vi "subDAQ_GetSnapPoint.vi"(5 "Record Table Refnum":refnum<vi>, 7 "Snap Number Refnum":refnum<vi>, 8 "Snap Point Y Arr Refnum":refnum<vi>, 9 "Snap Point X Arr Refnum":refnum<vi>, 10 "Snap Number Counting":dbl=2.0, 11 "Stage Status":T1={" Current Position"=[4.5511, -4.228, 0.0], "Number of Axis"=3, "ILSID"=1}) -> (1 "Snap Point cluster":cluster{"Snap Y":dbl[], "Snap X":dbl[]}={"Snap Y"=[-4.228, -2.7513], "Snap X"=[4.5511, 4.6806]}, 2 "Snap Point  Y Array":dbl[](array[numeric]), 3 "Snap Point  X Array":dbl[](array[numeric]))   [LabVIEW 2015]
panel:
  # "X"
  # "Y"
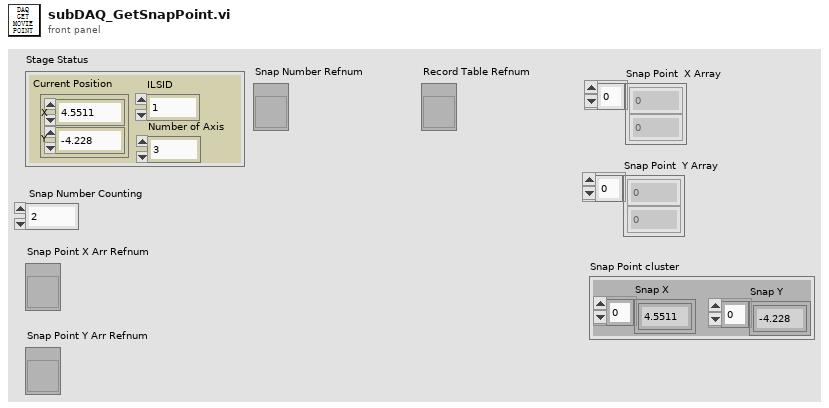
[diagram p1: front panel]
types:
  T1 = cluster{" Current Position":dbl[], "Number of Axis":i32, "ILSID":i32}
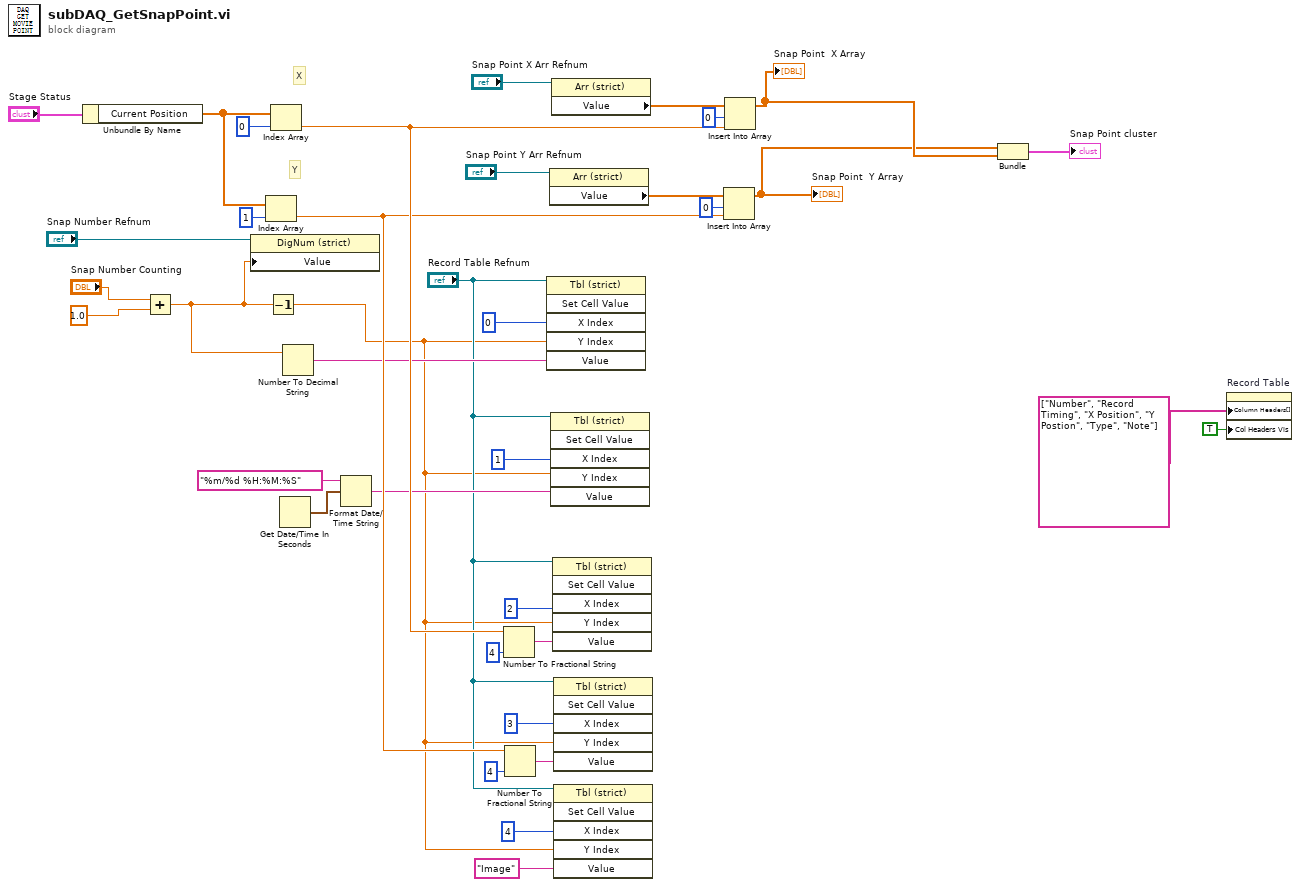
[diagram p0: block diagram]
diagram:
  # "Y"
  # "X"
  n1 = Unbundle By Name("Stage Status") -> ("Current Position"=w23:dbl[])
  n2 = Add(x="Snap Number Counting", y=1.0) -> (x+y=w4:dbl)
  n3 = property class="DigNum (strict)"(reference="Snap Number Refnum", "Value"=w4) -> ()  [unwired: 1 in, 2 out]
  n4 = Index Array(array=w23, index=1) -> (element=w26:dbl)
  n5 = Decrement(x=w4) -> (x-1=w3:dbl)
  n6 = Index Array(array=w23, index=0) -> (element=w27:dbl)
  n7 = Get Date/Time In Seconds() -> (seconds since 1Jan1904=w30:timestamp)
  n8 = Number To Decimal String(number=w4) -> (decimal integer string=w14:string)  [unwired: 1 in]
  n9 = Format Date/Time String(time format string (%c)="%m/%d %H:%M:%S", seconds (now)=w30) -> (date/time string=w12:string)  [unwired: 1 in]
  n10 = Number To Fractional String(number=w27, precision (6)=i16 4) -> (F-format string=w10:string)  [unwired: 2 in]
  n11 = Number To Fractional String(number=w26, precision (6)=i16 4) -> (F-format string=w8:string)  [unwired: 2 in]
  n12 = invoke class="Tbl (strict)" method="Set Cell Value"(reference="Record Table Refnum", "X Index"=0, "Y Index"=w3, "Value"=w14) -> ()  [unwired: 2 in, 6 out]
  n13 = property class="Arr (strict)"(reference="Snap Point Y Arr Refnum") -> ("Value"=w16:dbl[])  [unwired: 1 in, 2 out]
  n14 = invoke class="Tbl (strict)" method="Set Cell Value"(reference="Record Table Refnum", "X Index"=1, "Y Index"=w3, "Value"=w12) -> ()  [unwired: 2 in, 6 out]
  n15 = property class="Arr (strict)"(reference="Snap Point X Arr Refnum") -> ("Value"=w18:dbl[])  [unwired: 1 in, 2 out]
  n16 = invoke class="Tbl (strict)" method="Set Cell Value"(reference="Record Table Refnum", "X Index"=2, "Y Index"=w3, "Value"=w10) -> ()  [unwired: 2 in, 6 out]
  n17 = invoke class="Tbl (strict)" method="Set Cell Value"(reference="Record Table Refnum", "X Index"=3, "Y Index"=w3, "Value"=w8) -> ()  [unwired: 2 in, 6 out]
  n18 = invoke class="Tbl (strict)" method="Set Cell Value"(reference="Record Table Refnum", "X Index"=4, "Y Index"=w3, "Value"="Image") -> ()  [unwired: 2 in, 6 out]
  n19 = Insert Into Array(array=w16, index=0, new element=w26) -> (w32:dbl[])
  "Snap Point  Y Array" <- w32
  n20 = Insert Into Array(array=w18, index=0, new element=w27) -> (w33:dbl[])
  "Snap Point  X Array" <- w33
  n21 = Bundle("Value"=w32, "Value"=w33) -> (→"Snap Point cluster":cluster{"Value":dbl[], "Value":dbl[]})  [unwired: 1 in]
  n22 = property on="Record Table" class="Tbl (strict)"("Column Headers[]"=string[] ["Number", "Record Timing", "X Position", "Y Postion", "Type", "Note"] ("Column Header Strings[]"), "Col Headers Vis"=TRUE ("Visible Items:Column Headers Visible")) -> ()  [unwired: 2 in, 2 out]
